vi "Serialize - Text.vi"(8 "error in":errorcluster, 11 "TECData in":refnum<class "TECData.lvclass">) -> (0 "error out":errorcluster, 2 "Serialized Text":string, 3 "TECData out":refnum<class "TECData.lvclass">)   [LabVIEW 2014, in "TE Cooler.lvlib" / "TECData.lvclass"]
uses:
  TECData.lvclass
  TECData.lvclass/TECData.ctl
  reusable/Data/Data.lvclass
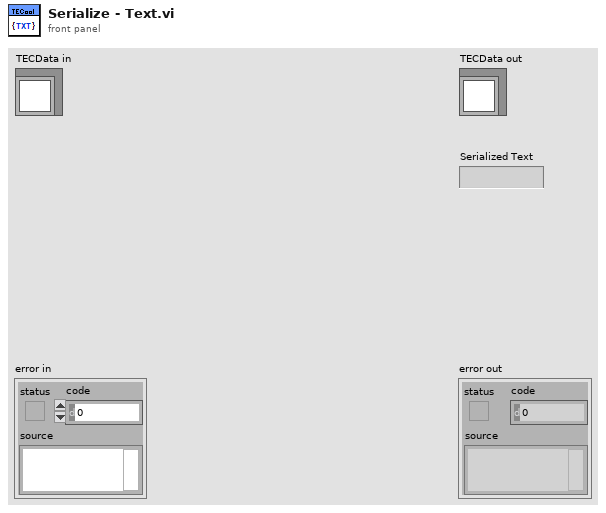
[diagram p1: front panel]
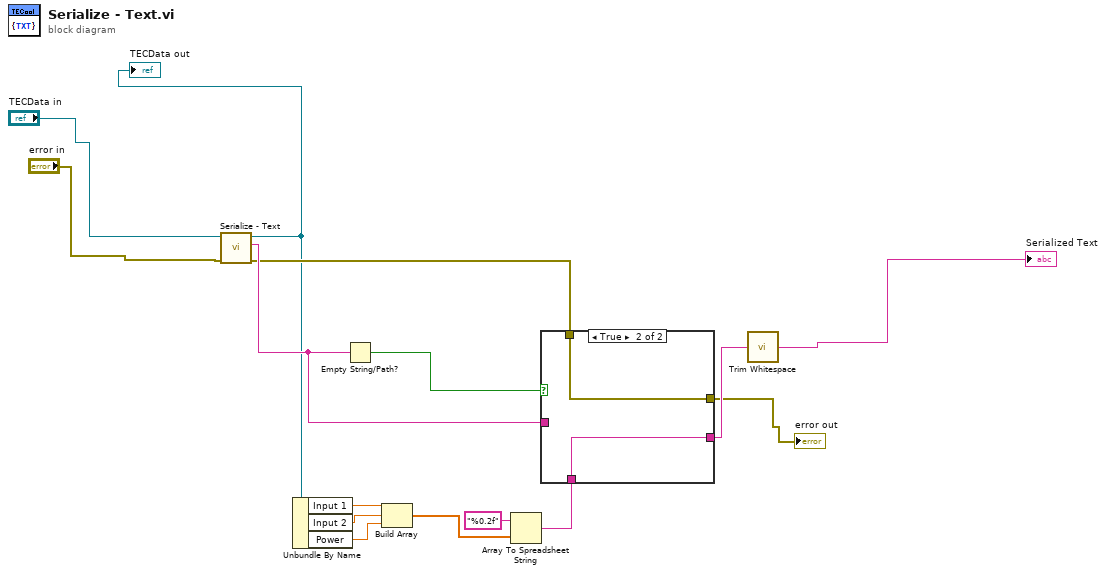
[diagram p0: block diagram]
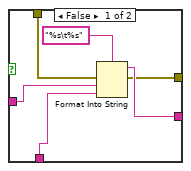
[diagram p2: hidden frame]
diagram:
  n1 = call-parent "Serialize - Text.vi"("error in"="error in", "Data in"="TECData in") -> ("error out"=w7:errorcluster, "Serialized Text"=w14:string, "Data out"=w4:refnum<class "TECData.lvclass">)  [unwired: 7 in]
  "TECData out" <- w4
  n2 = Unbundle By Name(w4) -> ("Input 1"=w13:sgl, "Input 2"=w12:sgl, "Power"=w11:sgl)
  n3 = Empty String/Path?(string/path=w14) -> (empty?=w15:bool)
  n4 = Build Array(w13, w12, w11) -> (w10:sgl[])
  n5 = Array To Spreadsheet String(array=w10, 3:"%0.2f" ("format string")) -> (spreadsheet string=w8:string)  [unwired: 1 in]
  n6 = case shown="True" w15 {
    tunnel: w14 -> [w20 _]
    tunnel: w8 -> [w19 w23]
    tunnel: [w18 w23] -> w6
    tunnel: w7 -> [w17 w22]
    tunnel: [w16 w22] -> w3
    frame False {
      n7 = Format Into String(format string="%s\t%s", error in=w17, w20, w19) -> (resulting string=w18:string, error out=w16:errorcluster)  [unwired: 1 in]
    }
    frame True {
    }
  }
  "error out" <- w3
  n8 = call <vilib>:"Trim Whitespace.vi"("string"=w6) -> ("trimmed string"=→"Serialized Text":string)  [unwired: 1 in]
